vi "Sine Graph.vi"() -> ()   [LabVIEW 2023]
panel:
  out "y":dbl
  out "x":dbl
  in  "n":dbl
  out "XY Graph":cluster{dbl[], dbl[]}(graph)
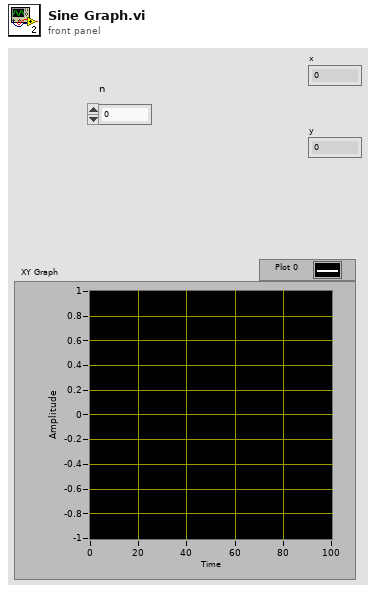
[diagram p1: front panel]
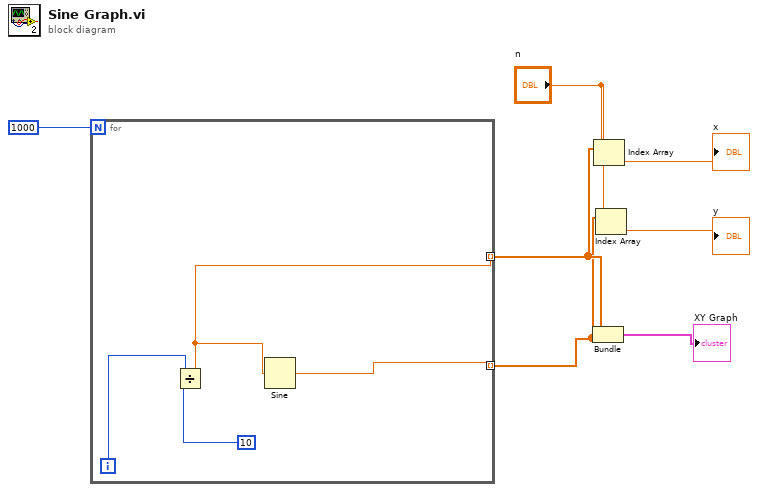
[diagram p0: block diagram]
diagram:
  n1 = for {
    N: 1000 -> [_]
    tunnel: [w11] -> w3 mode=indexing
    tunnel: [w8] -> w5 mode=indexing
    i -> [w10]
    n2 = Divide(x=w10, y=10) -> (x/y=w8:dbl)
    n3 = Sine(x=w8) -> (sin(x)=w11:dbl)
  }
  n4 = Bundle(w5, w3) -> (→"XY Graph":cluster{dbl[], dbl[]})  [unwired: 1 in]
  n5 = Index Array(array=w5, index="n") -> (element=→"x":dbl)
  n6 = Index Array(array=w3, index="n") -> (element=→"y":dbl)
